vi "Agilent PSG MXG Series Analog Modulation.vi"() -> ()   [LabVIEW 2018]
doc: "This example shows how to configure AM and FM.\n\n<b>Notes:</b>\n(1) This VI is NOT valid in E8247C.\n(2) For E8257D, E8267D, N5161A, N5162A, N5181A, N5182A, N5183A, N5171B, N5172B, N5181B, N5182B, N5173B, N5183B, this VI is valid only when the instrument installs <B>Option UNT</B>.\n(3) For N5171B, N5172B, N5181B, N5182B, N5173B, N5183B, only Modulation Type, Modulation Path and Modulation Source are valid."
uses:
  Agilent PSG MXG Series.lvlib
panel:
  in  "FM Modulation Source (2: External1)":u16(ring)=2 items=["Internal1", "Internal2", "External1", "External2", "Sweep", "Dual", "Noise1", "Noise2"]
  in  "AM Modulation Source (0: Internal1)":u16(ring) items=["Internal1", "Internal2", "External1", "External2", "Sweep", "Dual", "Noise1", "Noise2"]
  in  "VISA resource name":refnum<visa-resource-name>
  in  "Enable Deviation Coupling (T:Enable)":bool=TRUE
  in  "FM Deviation (1000 Hz)":dbl=1000.0
  in  "Enable Depth Coupling (T:Enable)":bool=TRUE
  in  "AM Type (0: Linear)":u16(ring) items=["Linear", "Exponential"]
  in  "AM Depth (10 percent)":dbl=10.0
  in  "FM Modulation Path (1)":u16(ring)=1 items=["1"=1, "2"=2]
  in  "AM Modulation Path (1)":u16(ring)=1 items=["1"=1, "2"=2]
  # "(c) 2007-2016 National Instruments.  ALL RIGHTS RESERVED."
  # "(1) This VI is NOT valid in E8247C.\n(2) For E8257D, E8267D, N5161A,  N5162A, N5181A, N5182A, N5183A, \nN5171B, N5172B, N5181B, N5182B, N5173B, N5183B,\nthis VI is valid only when the instrument installs Option UNT.\n(3) For N5171B, N5172B, N5181B, N5182B, N5173B, N5183B, \nonly Modulation Type, Modulation Path and Modulation Source are valid."
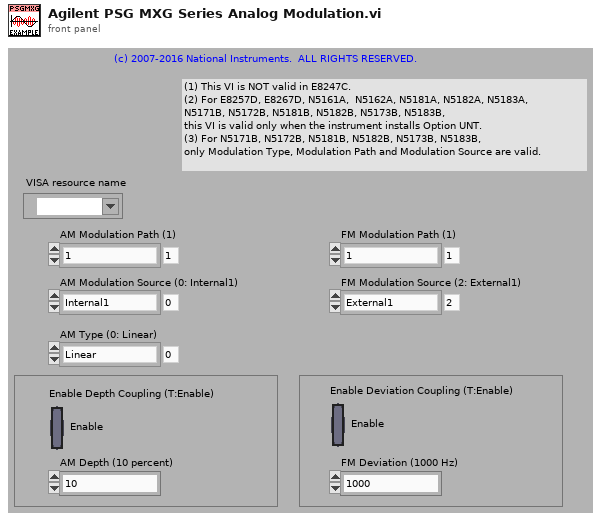
[diagram p1: front panel]
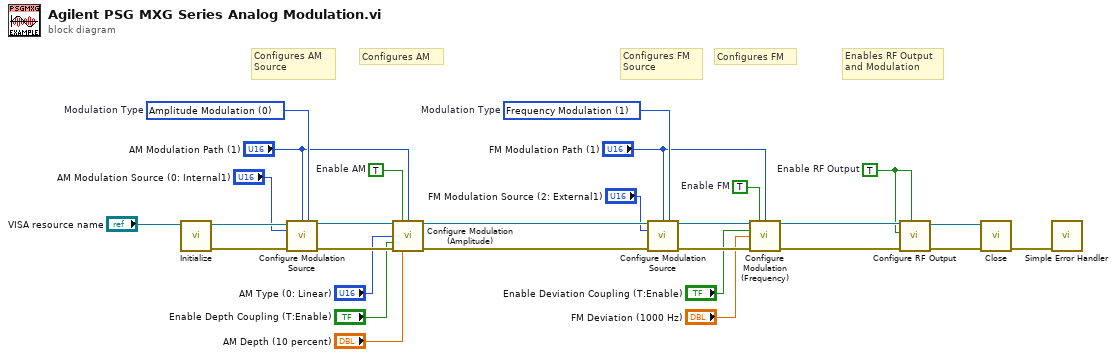
[diagram p0: block diagram]
diagram:
  w3 = TRUE  # Enable RF Output
  w17 = TRUE  # Enable FM
  w20 = u16 1 items=["Amplitude Modulation", "Frequency Modulation", "Phase Modulation"]  # Modulation Type
  w23 = TRUE  # Enable AM
  w28 = u16 0 items=["Amplitude Modulation", "Frequency Modulation", "Phase Modulation"]  # Modulation Type
  # "Enables RF Output\nand Modulation"
  # "Configures FM"
  # "Configures FM\nSource"
  # "Configures AM"
  # "Configures AM\nSource"
  n1 = call "Initialize.vi"("VISA resource name"="VISA resource name") -> ("error out"=w26:errorcluster, "VISA resource name out"=w27:refnum<visa-resource-name>)  [unwired: 3 in, 6 out]
  n2 = call "Configure Modulation Source.vi"("VISA resource name"=w27, "Modulation Path (1)"="AM Modulation Path (1)", "Modulation Type (0: Amplitude Modulation)"=w28, "Modulation Source (0: Internal1)"="AM Modulation Source (0: Internal1)", "error in (no error)"=w26) -> ("VISA resource name out"=w25:refnum<visa-resource-name>, "error out"=w24:errorcluster)  [unwired: 5 in, 4 out]
  n3 = call "Configure Modulation (Amplitude).vi"("VISA resource name"=w25, "Enable AM (T:Enable)"=w23, "AM Path (1)"="AM Modulation Path (1)", "AM Type (0: Linear)"="AM Type (0: Linear)", "Enable Depth Coupling (T:Enable)"="Enable Depth Coupling (T:Enable)", "error in (no error)"=w24, "AM Depth (10 percent)"="AM Depth (10 percent)") -> ("VISA resource name out"=w22:refnum<visa-resource-name>, "error out"=w21:errorcluster)  [unwired: 2 in, 5 out]
  n4 = call "Configure Modulation Source.vi"("VISA resource name"=w22, "Modulation Path (1)"="FM Modulation Path (1)", "Modulation Type (0: Amplitude Modulation)"=w20, "Modulation Source (0: Internal1)"="FM Modulation Source (2: External1)", "error in (no error)"=w21) -> ("VISA resource name out"=w16:refnum<visa-resource-name>, "error out"=w15:errorcluster)  [unwired: 5 in, 4 out]
  n5 = call "Configure Modulation (Frequency).vi"("VISA resource name"=w16, "Enable FM (T:Enable)"=w17, "FM Path (1)"="FM Modulation Path (1)", "Enable Deviation Coupling (T:Enable)"="Enable Deviation Coupling (T:Enable)", "FM Deviation (1000 Hz)"="FM Deviation (1000 Hz)", "error in (no error)"=w15) -> ("VISA resource name out"=w12:refnum<visa-resource-name>, "error out"=w11:errorcluster)  [unwired: 8 out]
  n6 = call "Configure RF Output.vi"("Enable Modulation (T:Enable)"=w3, "error in (no error)"=w11, "Enable RF Output (F:Disable)"=w3, "VISA resource name"=w12) -> ("error out"=w9:errorcluster, "VISA resource name out"=w10:refnum<visa-resource-name>)  [unwired: 4 in, 2 out]
  n7 = call "Close.vi"("error in (no error)"=w9, "VISA resource name"=w10) -> ("error out"=w8:errorcluster)  [unwired: 9 out]
  n8 = call <vilib>:"Simple Error Handler.vi"("error in (no error)"=w8) -> ()  [unwired: 1 in, 8 out]
